vi "MKS670_RS232_init.vi"(11 "VISA in":refnum<visa-resource-name>) -> (0 "error out":errorcluster, 3 "VISA out":refnum<visa-resource-name>, 4 "status":bool)   [LabVIEW 2019]
uses:
  <vilib>/Instr/_visa.llb/VISA Flush IO Buffer Mask.ctl
  <vilib>/Instr/_visa.llb/VISA Configure Serial Port (Instr).vi
panel:
  out "read buffer":string
  out "version":dbl
  out "Array":bool[](array[boolean])
  out "Error at VISA Read 6":errorcluster
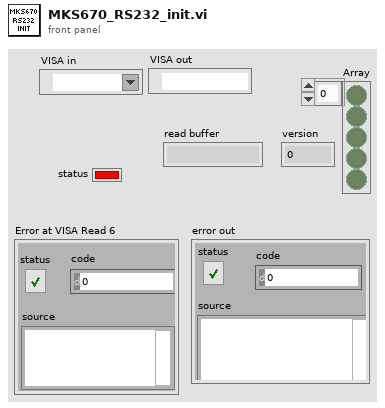
[diagram p1: front panel]
types:
  T1 = typedef "VISA Flush IO Buffer Mask.ctl" = u16
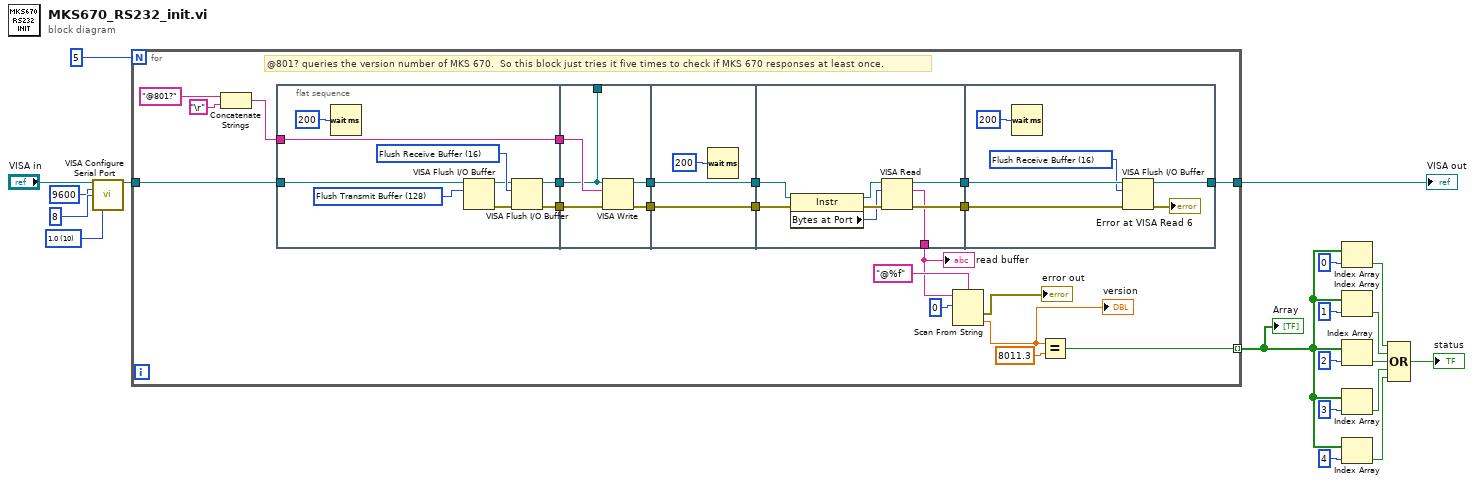
[diagram p0: block diagram]
diagram:
  w2 = u16 10 items=["1.0"=10, "1.5"=15, "2.0"=20] ("stop bits (10: 1 bit)")
  n1 = call-poly "VISA Configure Serial Port"("VISA resource name"="VISA in", "baud rate (9600)"=u32 9600, "data bits (8)"=u16 8, "stop bits (10: 1 bit)"=w2) -> ("VISA resource name out"=w17:refnum<visa-resource-name>)  [unwired: 10 in, 1 out]
  n2 = for {
    N: 5 -> [_]
    tunnel: w17 -> [w25]
    tunnel: [w24] -> w16 mode=indexing
    tunnel: [w20] -> w1
    # "@801? queries the version number of MKS 670.  So this block just tries it five times to check if MKS 670 responses at least once."
    n3 = Concatenate Strings("@801?" ("string"), "\r") -> (w21:string)
    n4 = flat-sequence {
      tunnel: w25 -> [w44]
      tunnel: w21 -> [w49]
      tunnel: [w49] -> w40
      tunnel: [w43] -> w39
      tunnel: [w42] -> w38
      tunnel: [w51] -> _
      tunnel: [w53] -> w37
      tunnel: [w52] -> w36
      tunnel: w40 -> [w54]
      tunnel: w39 -> [w51]
      tunnel: w38 -> [w50]
      tunnel: w37 -> [w56]
      tunnel: [w56] -> w35
      tunnel: w36 -> [w55]
      tunnel: [w55] -> w34
      tunnel: w35 -> [w62]
      tunnel: w34 -> [w61]
      tunnel: [w60] -> w33
      tunnel: [w59] -> w32
      tunnel: [w58] -> w26
      tunnel: w33 -> [w70]
      tunnel: w32 -> [w69]
      tunnel: [w66] -> w20
      frame #0 {
        w48 = T1 16 items=["Flush Receive Buffer"=16, "Write Transmit Buffer to Device"=32, "Flush Receive Buffer (No I/O)"=64, "Flush Transmit Buffer"=128] ("Mask")
        w45 = T1 128 items=["Flush Receive Buffer"=16, "Write Transmit Buffer to Device"=32, "Flush Receive Buffer (No I/O)"=64, "Flush Transmit Buffer"=128] ("Mask")
        n5 = Wait (ms)(milliseconds to wait=u32 200) -> ()  [unwired: 1 out]
        n6 = VISA Flush I/O Buffer(VISA resource name=w44, mask (16)=w45) -> (VISA resource name out=w46:refnum<visa-resource-name>, error out=w47:errorcluster)  [unwired: 1 in]
        n7 = VISA Flush I/O Buffer(VISA resource name=w46, mask (16)=w48, error in (no error)=w47) -> (VISA resource name out=w43:refnum<visa-resource-name>, error out=w42:errorcluster)
      }
      frame #1 {
        n8 = VISA Write(VISA resource name=w51, write buffer=w54, error in (no error)=w50) -> (VISA resource name out=w53:refnum<visa-resource-name>, error out=w52:errorcluster)  [unwired: 1 out]
      }
      frame #2 {
        n9 = Wait (ms)(milliseconds to wait=u32 200) -> ()  [unwired: 1 out]
      }
      frame #3 {
        n10 = property class="Instr"(reference=w62, error in=w61) -> (reference out=w63:refnum<visa-resource-name>, error out=w65:errorcluster, "Bytes at Port"=w64:u32)
        n11 = VISA Read(VISA resource name=w63, byte count=w64, error in (no error)=w65) -> (VISA resource name out=w60:refnum<visa-resource-name>, read buffer=w58:string, error out=w59:errorcluster)  [unwired: 1 out]
      }
      frame #4 {
        w67 = T1 16 items=["Flush Receive Buffer"=16, "Write Transmit Buffer to Device"=32, "Flush Receive Buffer (No I/O)"=64, "Flush Transmit Buffer"=128] ("Mask")
        n12 = Wait (ms)(milliseconds to wait=u32 200) -> ()  [unwired: 1 out]
        n13 = VISA Flush I/O Buffer(VISA resource name=w70, mask (16)=w67, error in (no error)=w69) -> (VISA resource name out=w66:refnum<visa-resource-name>, error out=→"Error at VISA Read 6":errorcluster)
      }
    }
    n14 = Scan From String(format string="@%f", input string=w26, initial scan location=u32 0) -> (error out=→"error out":errorcluster, output 1=w28:dbl)  [unwired: 2 in, 2 out]
    "version" <- w28
    n15 = Equal?(x=w28, y=8011.3) -> (x = y?=w24:bool)
    "read buffer" <- w26
  }
  "Array" <- w16
  "VISA out" <- w1
  n16 = Index Array(array=w16, index=0) -> (element=w12:bool)
  n17 = Index Array(array=w16, index=1) -> (element=w11:bool)
  n18 = Index Array(array=w16, index=2) -> (element=w13:bool)
  n19 = Index Array(array=w16, index=3) -> (element=w14:bool)
  n20 = Index Array(array=w16, index=4) -> (element=w15:bool)
  n21 = Compound Arithmetic op=OR(w12, w11, w13, w14, w15) -> (→"status":bool)
